vi "Read EnFlo Tunnel RPM.vi"() -> ()   [LabVIEW 2021]
uses:
  ADAM Client/Sub VIs/ADAM Controls/Update_scan_value.ctl
  ADAM_Global.vi
  <vilib>/Analysis/NI_AALBase.lvlib
panel:
  out "EnFlo Tunnel Motor Enabled":bool
  in  "rate":dbl=20000.0
  in  "stop":bool
  in  "number of samples":i32=200000
  out "St Dev":dbl[](array[numeric])
  out "Mean":dbl[](array[numeric])
  out "Waveform Graph":dbl[][](graph)
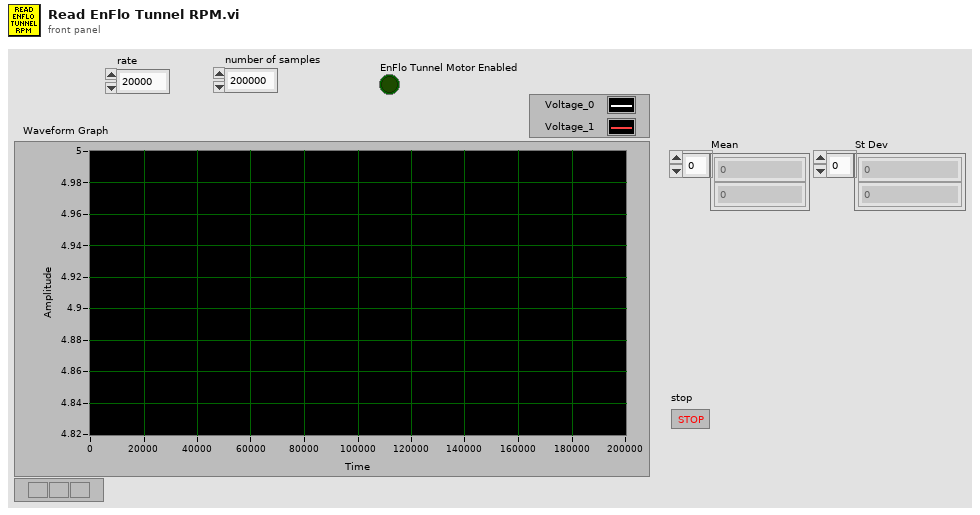
[diagram p1: front panel]
types:
  T1 = enum16{"Append to Global", "Read Global then Clear"}
  T2 = typedef "Update_scan_value.ctl" = cluster{"Channel Name":string, "New Value":dbl, "!Auto_Off":bool}
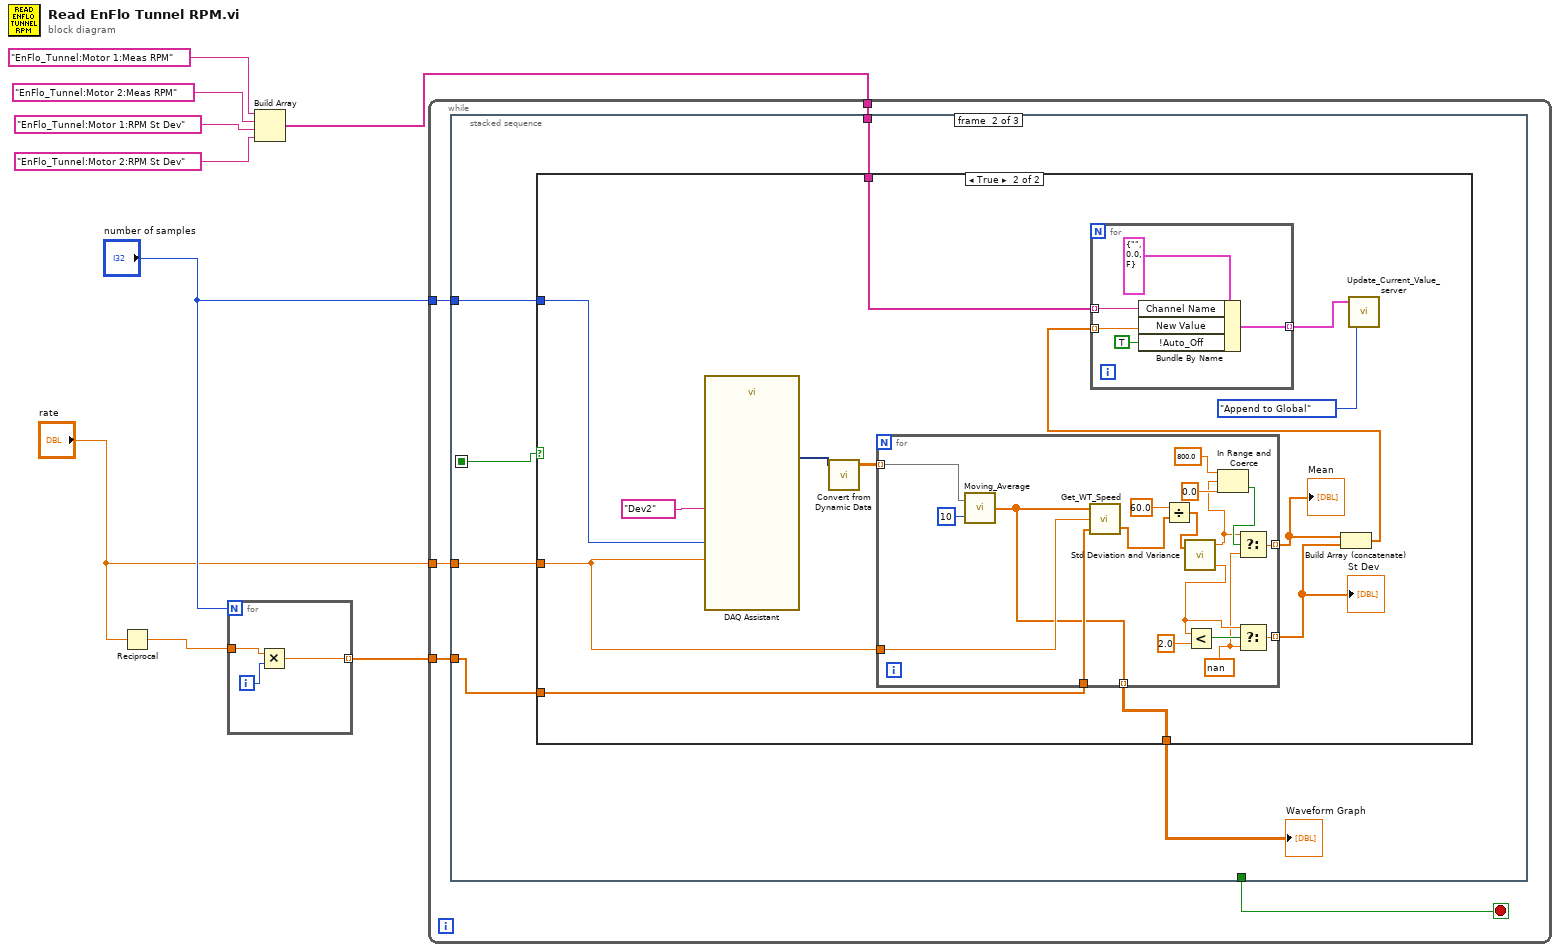
[diagram p0: block diagram]
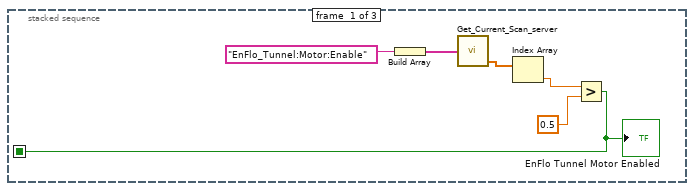
[diagram p2: hidden frame]
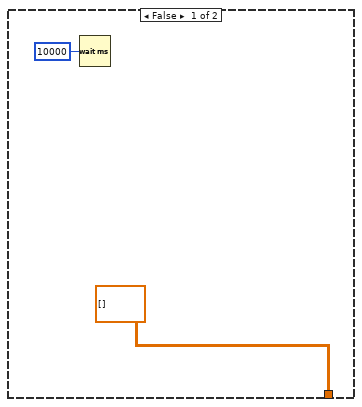
[diagram p3: hidden frame]
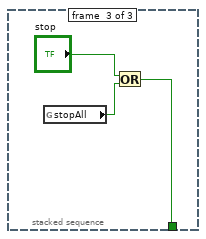
[diagram p4: hidden frame]
diagram:
  n1 = Reciprocal(x="rate") -> (1/x=w9:dbl)
  n2 = for {
    N: "number of samples" -> [_]
    tunnel: w9 -> [w12]
    tunnel: [w10] -> w8 mode=indexing
    i -> [w11]
    n3 = Multiply(x=w12, y=w11) -> (x*y=w10:dbl)
  }
  n4 = Build Array("EnFlo_Tunnel:Motor 1:Meas RPM", "EnFlo_Tunnel:Motor 2:Meas RPM", "EnFlo_Tunnel:Motor 1:RPM St Dev", "EnFlo_Tunnel:Motor 2:RPM St Dev") -> (w4:string[])
  n5 = while {
    tunnel: w8 -> [w17]
    tunnel: "rate" -> [w16]
    tunnel: "number of samples" -> [w15]
    tunnel: w4 -> [w14]
    stop <- w13 stop-if-true
    n6 = stacked-sequence {
      seq-local: [w18 _ _] -> [_ w24 _]
      tunnel: w17 -> [_ w29 _]
      tunnel: w16 -> [_ w28 _]
      tunnel: w15 -> [_ w27 _]
      tunnel: w14 -> [_ w26 _]
      tunnel: [_ _ w68] -> w13
      frame #0 {
        n7 = Build Array("EnFlo_Tunnel:Motor:Enable") -> (w22:string[])
        n8 = call "Get_Current_Scan_server.vi"("Desired Channels"=w22) -> ("Numerical Values"=w21:dbl[])  [unwired: 2 out]
        n9 = Index Array(array=w21) -> (element=w20:dbl)  [unwired: 1 in]
        n10 = Greater?(x=w20, y=0.5) -> (0:w18:bool)
        "EnFlo Tunnel Motor Enabled" <- w18
      }
      frame #1 {
        n11 = case shown="True" w24 {
          tunnel: w29 -> [_ w43]
          tunnel: w28 -> [_ w41]
          tunnel: w27 -> [_ w40]
          tunnel: w26 -> [_ w35]
          tunnel: [dbl[][] [] ("N+1-Period") w32] -> w25
          frame False {
            n12 = Wait (ms)(milliseconds to wait=u32 10000) -> ()  [unwired: 1 out]
          }
          frame True {
            n13 = call "DAQ Assistant"("rate"=w41, "number of samples"=w40, "device name"=tag "Dev2") -> ("data"=w39:dynamicdata)  [unwired: 14 in, 2 out]
            n14 = call "Convert from Dynamic Data"("Dynamic Data Type"=w39) -> ("Array"=w44:dbl[][])  [unwired: 3 in]
            n15 = for {
              tunnel: w44 -> [w66] mode=indexing
              tunnel: w41 -> [w65]
              tunnel: w43 -> [w64]
              tunnel: [w50] -> w38 mode=indexing
              tunnel: [w56] -> w37 mode=indexing
              tunnel: [w60] -> w32 mode=indexing
              w52 = nan
              n16 = call "Moving_Average.vi"("Period"=10, "Input Array"=w66) -> ("N+1-Period"=w60:dbl[])
              n17 = call "Get_WT_Speed.vi"("Time (s)"=w64, "Av Sampling Rate"=w65, "Opto Trace"=w60) -> ("Time per Cycle"=w62:dbl[])  [unwired: 1 out]
              n18 = Divide(x=60.0, y=w62) -> (x/y=w61:dbl[])
              n19 = call <vilib>:"Std Deviation and Variance.vi"("X"=w61) -> ("mean"=w51:dbl, "variance"=w57:dbl)  [unwired: 1 in, 1 out]
              n20 = Less?(x=w57, y=2.0) -> (x < y?=w58:bool)
              n21 = In Range and Coerce(upper limit=800.0, x=w51, lower limit=0.0) -> (In Range?=w53:bool)  [unwired: 1 out]
              n22 = Select(t=w51, s=w53, f=w52) -> (s? t:f=w50:dbl)
              n23 = Select(t=w57, s=w58, f=w52) -> (s? t:f=w56:dbl)
            }
            "Mean" <- w38
            "St Dev" <- w37
            n24 = Build Array (concatenate)(w38, w37) -> (w36:dbl[])
            n25 = for {
              tunnel: w36 -> [w47] mode=indexing
              tunnel: w35 -> [w46] mode=indexing
              tunnel: [w45] -> w34 mode=indexing
              n26 = Bundle By Name(cluster=T2 {"Channel Name"="", "New Value"=0.0, "!Auto_Off"=FALSE} ("Update Scan Value Cluster"), "Channel Name"=w46, "New Value"=w47, "!Auto_Off"=TRUE) -> (w45:T2)
            }
            n27 = call "Update_Current_Value_server.vi"("Mode"=T1."Append to Global", "Update array in"=w34) -> ()  [unwired: 1 in, 1 out]
          }
        }
        "Waveform Graph" <- w25
      }
      frame #2 {
        n28 = global read "ADAM_Global.vi" "stopAll"() -> (w69:bool)
        n29 = Or(x="stop", y=w69) -> (x .or. y?=w68:bool)
      }
    }
  }
